vi "getPressure.vi"(6 "Channel":i32, 8 "error in (no error)":errorcluster, 11 "Instrument.Cryostat in":refnum<class "Instrument.Cryostat.lvclass">) -> (0 "error out":errorcluster, 1 "Status":string, 2 "Pressure (mbar)":dbl, 3 "Instrument.Cryostat out":refnum<class "Instrument.Cryostat.lvclass">)   [LabVIEW 2019, in "Instrument.Cryostat.lvclass"]
uses:
  Instrument.Cryostat.lvclass
  Typedefs/getPressure--cluster.ctl
  Typedefs/Cryostat.commands--enum.ctl
  e0c1ba74-9f4c-489b-94fc-669e0b58d831.vi
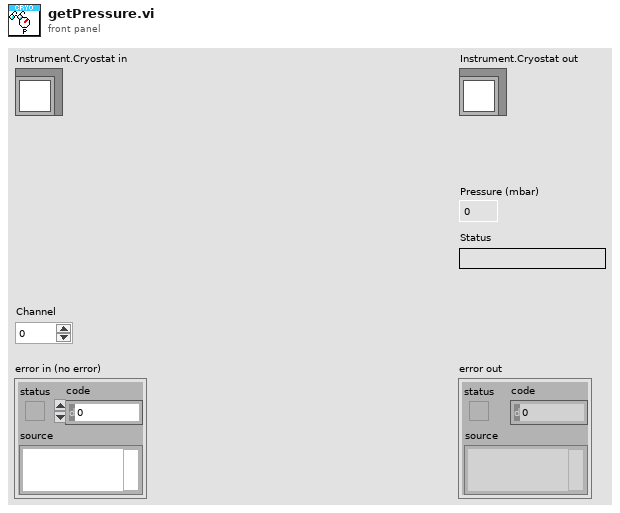
[diagram p1: front panel]
types:
  T1 = typedef "Instrument.Cryostat.lvclass/Cryostat.commands--enum.ctl" = enum16{"getLN2Level", "getLHeLevel", "getMagnet", "getMagnetVector", "setMagnet", "setMagnetVector", "getAngle", "setAngle", "getTemperature", "setTemperature", "getHeater", "setHeater", "getChamber", "setChamber", "getPressure"}
  T2 = typedef "Instrument.Cryostat.lvclass/getPressure--cluster.ctl" = cluster{"pressure":dbl, "status":string}
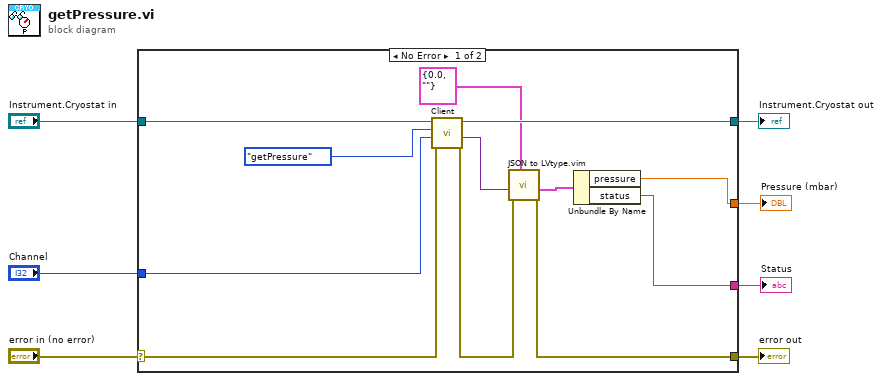
[diagram p0: block diagram]
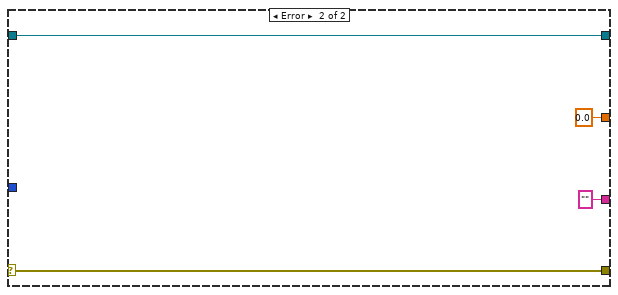
[diagram p2: hidden frame]
diagram:
  n1 = case shown="No Error" "error in (no error)" {
    selector: "error in (no error)" -> [w13 w23]
    tunnel: [w8 w23] -> w6
    tunnel: [w19 w22] -> w4
    tunnel: "Instrument.Cryostat in" -> [w14 w22]
    tunnel: "Channel" -> [w18 _]
    tunnel: [w17 0.0 ("Pressure")] -> w2
    tunnel: [w16 "" ("Status")] -> w1
    frame No Error {
      n2 = call-dynamic "Client.vi"("error in (no error)"=w13, "Data in"=w18, "Command in"=Cryostat.commands--enum."getPressure" ("commands"), "Instrument in"=w14) -> ("error out"=w10:errorcluster, "Data out"=w11:variant, "Instrument out"=w19:refnum<class "Instrument.Cryostat.lvclass">)  [unwired: 4 in, 1 out]
      n3 = call "JSON to LVtype.vim"("type"=T2 {"pressure"=0.0, "status"=""} ("getPressure"), "error in (no error)"=w10, "JSON Data in"=w11) -> ("error out"=w8:errorcluster, "Data out"=w9:T2)  [unwired: 7 in]
      n4 = Unbundle By Name(w9) -> ("pressure"=w17:dbl, "status"=w16:string)
    }
    frame Error {
    }
  }
  "error out" <- w6
  "Instrument.Cryostat out" <- w4
  "Pressure (mbar)" <- w2
  "Status" <- w1
